vi "AH_OPEN.vi"(8 "error in (no error)":errorcluster, 10 "Configuration Cluster":T1={"General"={"Config.ini"=path "", "Default Logging Path"=path ""}, "Hardware"={"Measure Rate (1/s)"=0, "HP DMM VISA"="", "LS 335 VISA"="", "HP DM"={"Range"=enum."Autorange", "Autozero"=FALSE, "Display"=enum."3 1/2 Digit", "Blank LCD"=FALSE}}, "Operation"={"Operation Mode"=enum."Idle-Off", "Status"="", "NewLog?"=FALSE, "OvenWarn"=FALSE}}) -> (0 "error out":errorcluster, 2 "Configuration Cluster Out":T1={"General"={"Config.ini"=path "", "Default Logging Path"=path ""}, "Hardware"={"Measure Rate (1/s)"=0, "HP DMM VISA"="", "LS 335 VISA"="", "HP DM"={"Range"=enum."Autorange", "Autozero"=FALSE, "Display"=enum."3 1/2 Digit", "Blank LCD"=FALSE}}, "Operation"={"Operation Mode"=enum."Idle-Off", "Status"="", "NewLog?"=FALSE, "OvenWarn"=FALSE}})   [LabVIEW 2021]
uses:
  Config_Cluster.ctl
  Mode_Enum.ctl
  <vilib>/Instr/_visa.llb/VISA Open Access Mode.ctl
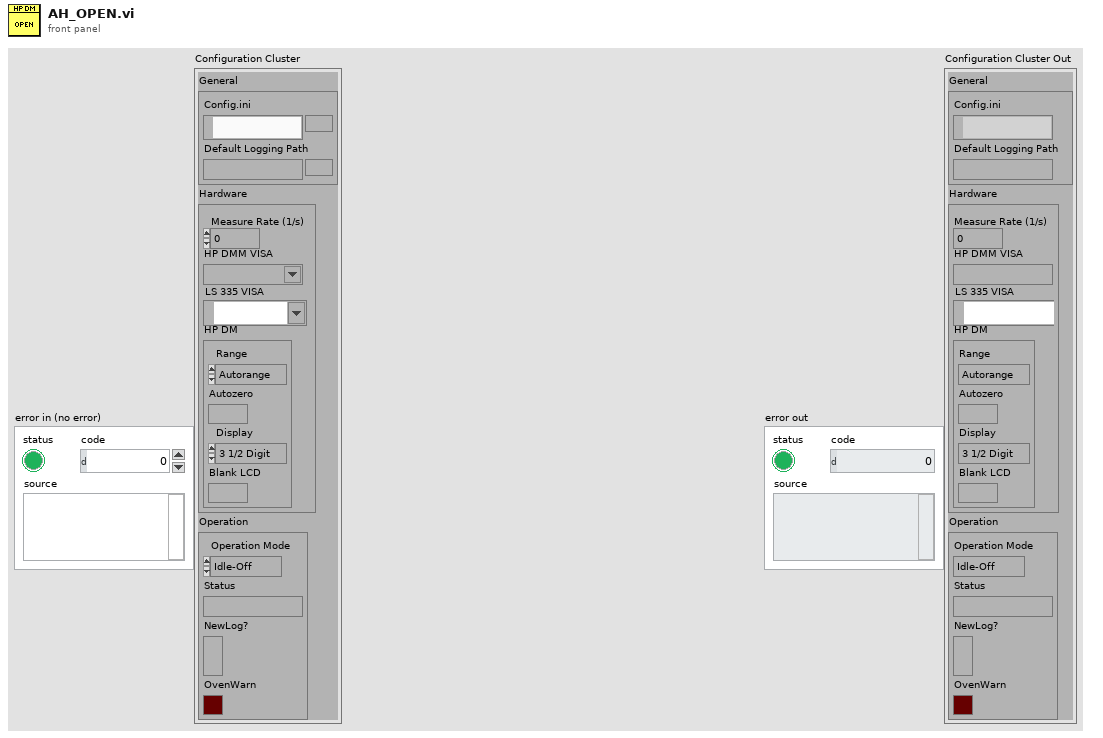
[diagram p1: front panel]
types:
  T1 = typedef "Config_Cluster.ctl" = cluster{"General":cluster{"Config.ini":path, "Default Logging Path":path}, "Hardware":cluster{"Measure Rate (1/s)":i32, "HP DMM VISA":refnum<visa-resource-name>, "LS 335 VISA":refnum<visa-resource-name>, "HP DM":cluster{"Range":enum16{"Autorange", "30mV", "300mV", "3V", "30V"}, "Autozero":bool, "Display":enum16{"3 1/2 Digit", "4 1/2 Digit", "5 1/2 Digit"}, "Blank LCD":bool}}, "Operation":cluster{"Operation Mode":T2, "Status":string, "NewLog?":bool, "OvenWarn":bool}}
  T2 = typedef "Mode_Enum.ctl" = enum16{"OvenNRDY", "Logging", "Idle-Off", "Idle"}
  T3 = typedef "VISA Open Access Mode.ctl" = u32
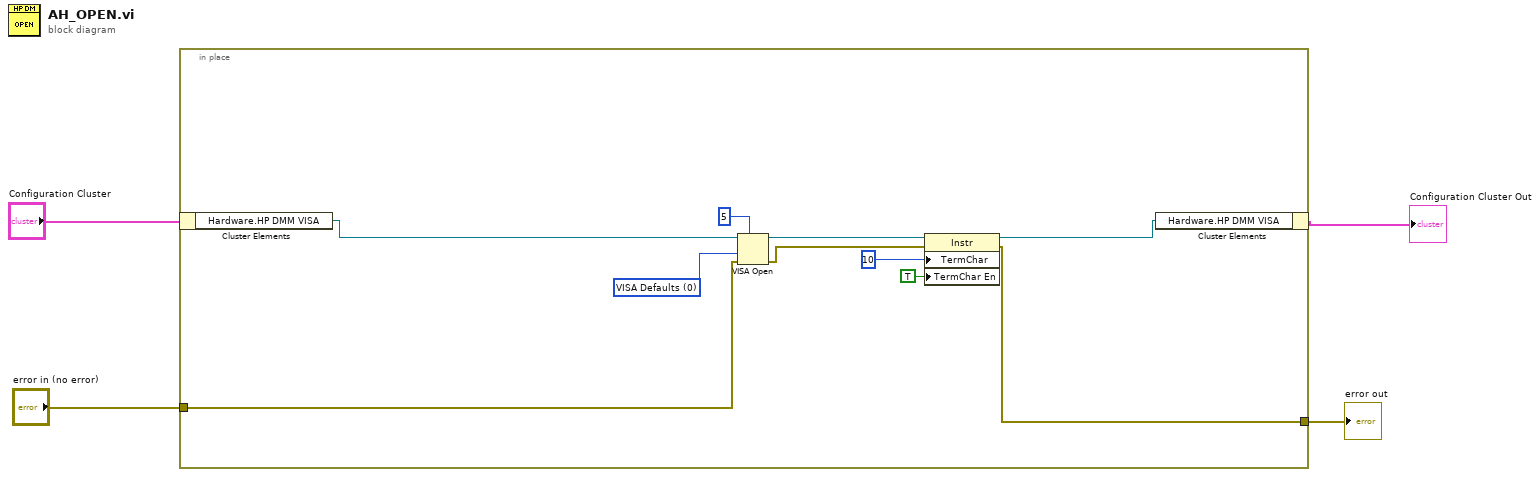
[diagram p0: block diagram]
diagram:
  n1 = in-place {
    in-place-border: "error in (no error)" -> [w12]
    in-place-border: [w7] -> w3
    w13 = T3 0 items=["VISA Defaults"=0, "Exclusive Lock"=1, "Load Configured Settings"=4] ("Access Mode")
    n2 = in-place-cluster #1("Configuration Cluster") -> ("Hardware.HP DMM VISA"=w11:refnum<visa-resource-name>)
    n3 = VISA Open(timeout (0)=u32 5 ("VISA Open timeout (0)"), access mode=w13, error in (no error)=w12, VISA resource name=w11) -> (VISA resource name=w10:refnum<visa-resource-name>, error out=w8:errorcluster)  [unwired: 1 in]
    n4 = property class="Instr"(reference=w10, error in=w8, "TermChar"=u8 10 ("Message Based Settings:Termination Character"), "TermChar En"=TRUE ("Message Based Settings:Termination Character Enable")) -> (reference out=w9:refnum<visa-resource-name>, error out=w7:errorcluster)
    n5 = in-place-cluster #1("Hardware.HP DMM VISA"=w9) -> (→"Configuration Cluster Out":T1)
  }
  "error out" <- w3
